vi "Initialize.vi"(8 "error in (no error)":errorcluster) -> (0 "error out":errorcluster, 3 "GCentral API out":refnum<class "GCentral API.lvclass">)   [LabVIEW 2020, in "GCentral-API.lvlib" / "GCentral API.lvclass"]
uses:
  GCentral API.lvclass
  GCentral API.lvclass/GCentral API.ctl
  GCentral-API.lvlib
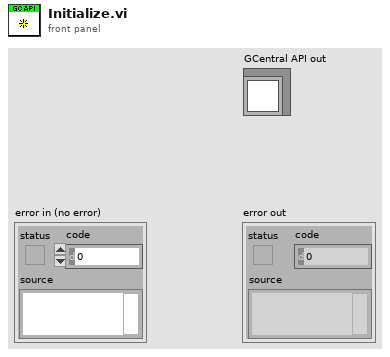
[diagram p1: front panel]
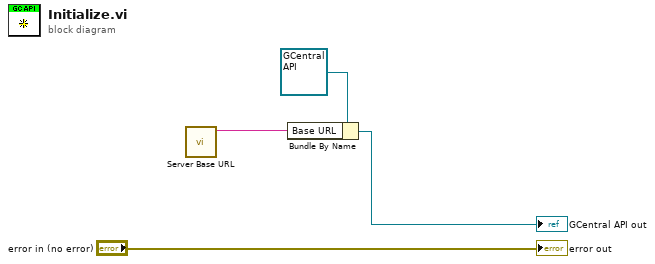
[diagram p0: block diagram]
diagram:
  n1 = call "Server Base URL.vi"() -> ("Server Base URI"=w1:string)  [unwired: 11 in]
  n2 = Bundle By Name(cluster=refnum<class "GCentral API.lvclass"> refnum ("GCentral API in"), "Base URL"=w1) -> (→"GCentral API out":refnum<class "GCentral API.lvclass">)
  "error out" <- "error in (no error)"
